vi "fgt read Ttl.vi"(8 "error in (no error)":errorcluster, 11 "TtlIndex":u32) -> (0 "error out":errorcluster, 3 "state out":bool)   [LabVIEW 2020, in "fgt_SDK.lvlib"]
doc: "Read TTL ports (BNC ports) if set as input."
uses:
  fgt_SDK.lvlib
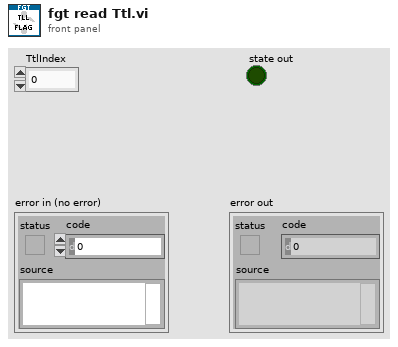
[diagram p1: front panel]
types:
  T1 = typedef "fgt_SDK.lvlib/fgt_STATUS_INFO.ctl" = cluster{"InstrType":T2, "instrSN":u16, "errorCode":u8, "infoCode":u8, "detail":string}
  T2 = typedef "fgt_SDK.lvlib/fgt_INSTRUMENT_TYPE.ctl" = enum32{"None", "MFCS", "MFCS_EZ", "FRP", "LineUP", "IPS"}
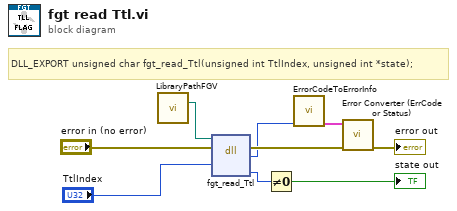
[diagram p0: block diagram]
diagram:
  # "DLL_EXPORT unsigned char fgt_read_Ttl(unsigned int TtlIndex, unsigned int *state);"
  n1 = call "LibraryPathFGV.vi"() -> ("Path Out"=w1:path)  [unwired: 14 in, 1 out]
  n2 = dll-call lib="C:/Workspace/fgt-SDK/LabVIEW/dlls/fgt_SDK_*.*" fn="fgt_read_Ttl"(path in=w1, error in="error in (no error)", "TtlIndex"="TtlIndex") -> (error out=w6:errorcluster, "return type"=w4:u8, "state"=w8:u32)  [unwired: 3 in, 1 out]
  n3 = Not Equal To 0?(x=w8) -> (x != 0?=→"state out":bool)
  n4 = call "ErrorCodeToErrorInfo.vi"("return type"=w4) -> ("StatusInfo"=w3:T1)  [unwired: 10 in]
  n5 = call "Error Converter (ErrCode or Status).vi"("error in (no error)"=w6, "StatusInfo"=w3) -> ("error out"=→"error out":errorcluster)  [unwired: 9 in]
